vi "PLC.CheckError.vi"(8 "error in (no error)":errorcluster, 10 "Result":i32) -> (0 "error out":errorcluster)   [LabVIEW 2016]
uses:
  Snap7/lib/Snap7.lvlib
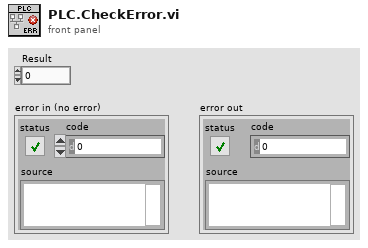
[diagram p1: front panel]
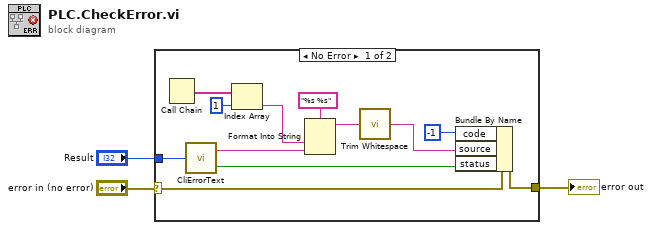
[diagram p0: block diagram]
diagram:
  n1 = case shown="No Error" "error in (no error)" {
    selector: "error in (no error)" -> [w14 w16]
    tunnel: "Result" -> [w15 _]
    tunnel: [w11 w16] -> w3
    frame No Error {
      n2 = Call Chain() -> (call chain=w10:string[])
      n3 = call "CliErrorText.vi"("ErrNo"=w15) -> ("Error"=w13:bool, "ErrMessage"=w8:string)
      n4 = Index Array(array=w10, index=1) -> (element=w7:string)
      n5 = Format Into String(format string="%s %s", w7, w8) -> (resulting string=w5:string)  [unwired: 2 in, 1 out]
      n6 = call <vilib>:"Trim Whitespace.vi"("string"=w5) -> ("trimmed string"=w4:string)  [unwired: 1 in]
      n7 = Bundle By Name(cluster=w14, "code"=-1, "source"=w4, "status"=w13) -> (w11:errorcluster)
    }
    frame Error {
    }
  }
  "error out" <- w3
